vi "Caraya Time Measurement.vi"(9 "No. of Runs":i32=1, 10 "Test Cases":bool[](array[boolean])=[FALSE, FALSE, FALSE], 11 "All Test":bool=TRUE) -> (2 "Caraya report":string, 3 "ICov Testing time (seconds)":dbl)   [LabVIEW 2018]
panel:
  # "Caraya"
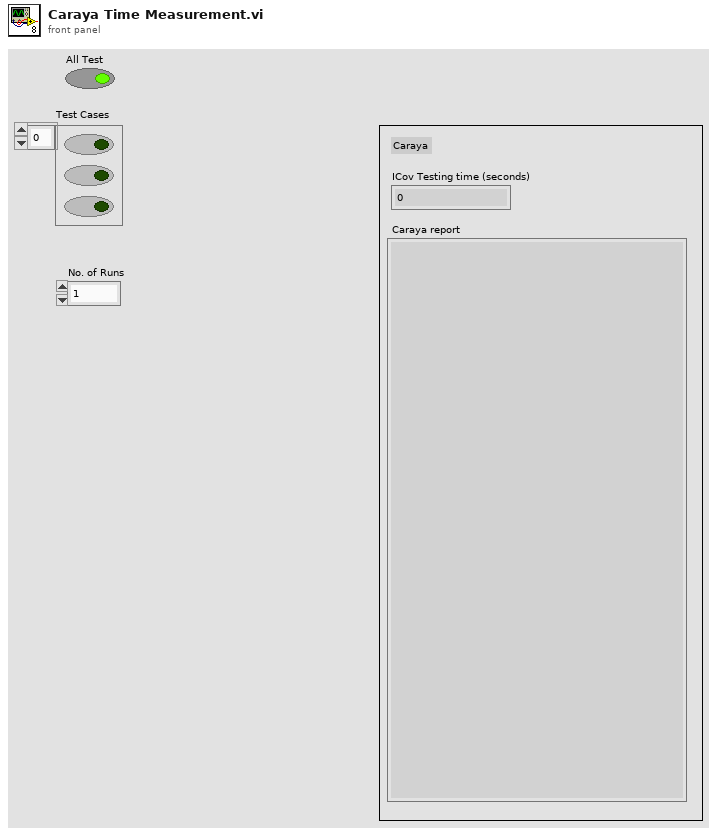
[diagram p1: front panel]
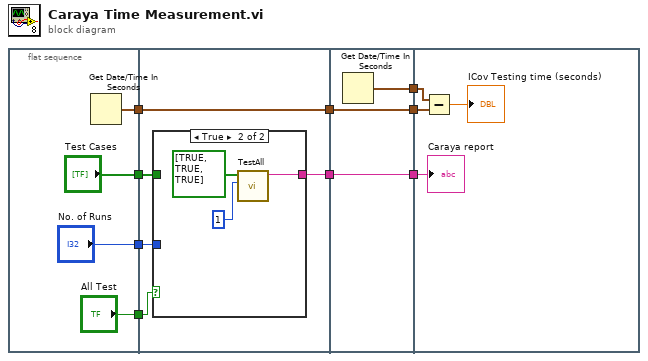
[diagram p0: block diagram]
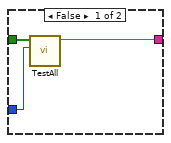
[diagram p2: hidden frame]
diagram:
  n1 = flat-sequence {
    tunnel: [w13] -> w9
    tunnel: ["Test Cases"] -> w3
    tunnel: ["All Test"] -> w2
    tunnel: ["No. of Runs"] -> w1
    tunnel: [w18] -> w8
    tunnel: w9 -> [w18]
    tunnel: [w17] -> w4
    tunnel: w3 -> [w16]
    tunnel: w2 -> [w15]
    tunnel: w1 -> [w14]
    tunnel: [w27] -> w7
    tunnel: [w26] -> w6
    tunnel: w8 -> [w26]
    tunnel: [w25] -> w5
    tunnel: w4 -> [w25]
    tunnel: w7 -> [w29]
    tunnel: w6 -> [w30]
    tunnel: w5 -> [w28]
    frame #0 {
      n2 = Get Date/Time In Seconds() -> (seconds since 1Jan1904=w13:timestamp)
    }
    frame #1 {
      n3 = case shown="True" w15 {
        tunnel: [w20 w24] -> w17
        tunnel: w16 -> [w21 _]
        tunnel: w14 -> [w19 _]
        frame False {
          n4 = call "TestAll.vi"("No. of Runs"=w19, "Test Cases"=w21) -> ("report"=w20:string)  [unwired: 8 in, 1 out]
        }
        frame True {
          n5 = call "TestAll.vi"("No. of Runs"=1, "Test Cases"=bool[] [TRUE, TRUE, TRUE]) -> ("report"=w24:string)  [unwired: 8 in, 1 out]
        }
      }
    }
    frame #2 {
      n6 = Get Date/Time In Seconds() -> (seconds since 1Jan1904=w27:timestamp)
    }
    frame #3 {
      n7 = Subtract(x=w29, y=w30) -> (x-y=→"ICov Testing time (seconds)":dbl)
      "Caraya report" <- w28
    }
  }
